vi "Combustion Calculations SubVI for 6.3a.vi"(1 "Array of Thermal Powers":dbl[](array[numeric]), 2 "Array of Fuel Flowrate":dbl[](array[numeric]), 3 "Array of (Fuel Flow * AFR)":dbl[](array[numeric]), 4 "Array of Air Flowrates":dbl[](array[numeric])) -> (0 "Driving Variables 2":T1)   [LabVIEW 2018]
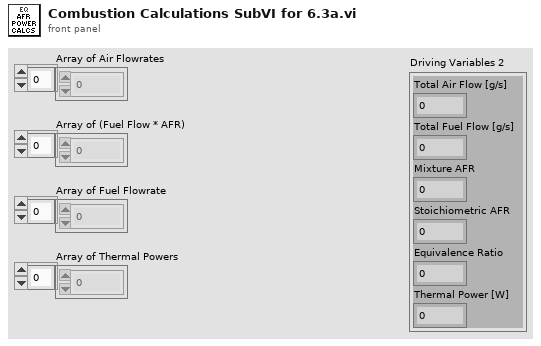
[diagram p1: front panel]
types:
  T1 = cluster{"Total Air Flow [g/s]":dbl, "Total Fuel Flow [g/s]":dbl, "Mixture AFR":dbl, "Stoichiometric AFR":dbl, "Equivalence Ratio":dbl, "Thermal Power [W]":dbl}
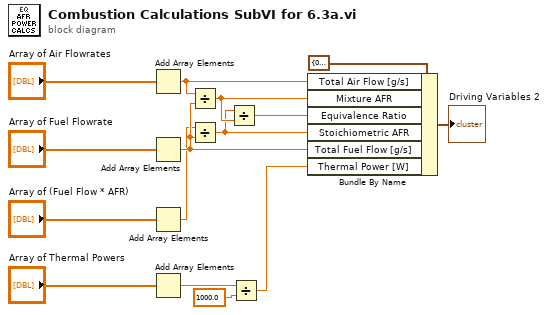
[diagram p0: block diagram]
diagram:
  n1 = Add Array Elements(numeric array="Array of Air Flowrates") -> (sum=w9:dbl)
  n2 = Add Array Elements(numeric array="Array of Fuel Flowrate") -> (sum=w8:dbl)
  n3 = Add Array Elements(numeric array="Array of (Fuel Flow * AFR)") -> (sum=w6:dbl)
  n4 = Add Array Elements(numeric array="Array of Thermal Powers") -> (sum=w13:dbl)
  n5 = Divide(x=w9, y=w8) -> (x/y=w12:dbl)
  n6 = Divide(x=w6, y=w8) -> (x/y=w11:dbl)
  n7 = Divide(x=w11, y=w12) -> (x/y=w10:dbl)
  n8 = Divide(x=w13, y=1000.0) -> (x/y=w15:dbl)
  n9 = Bundle By Name(cluster=T1 {"Total Air Flow [g/s]"=0.0, "Total Fuel Flow [g/s]"=0.0, "Mixture AFR"=0.0, "Stoichiometric AFR"=0.0, "Equivalence Ratio"=0.0, "Thermal Power [W]"=0.0} ("Driving Variables 2"), "Total Air Flow [g/s]"=w9, "Mixture AFR"=w12, "Equivalence Ratio"=w10, "Stoichiometric AFR"=w11, "Total Fuel Flow [g/s]"=w8, "Thermal Power [W]"=w15) -> (→"Driving Variables 2":T1)
